vi "flattenVelocityToXML_Scalar.vi"(8 "error in (no error)":errorcluster, 9 "velocityUnitInXML":T1, 10 "velocityAgain":variant, 11 "velocity":dbl[unit]) -> (0 "error out":errorcluster, 3 "xmlString":string)   [LabVIEW 2016, in "UnitsAndXML.lvlib"]
uses:
  <userlib>/Common/UnitsAndXML/UnitsAndXML.lvlib
  <userlib>/Common/UnitsAndXML/FlattenItemWithUnitToXML/FlattenVelocityToXML/VelocityUnit.ctl
  <vilib>/Utility/VariantDataType/VariantType.lvlib
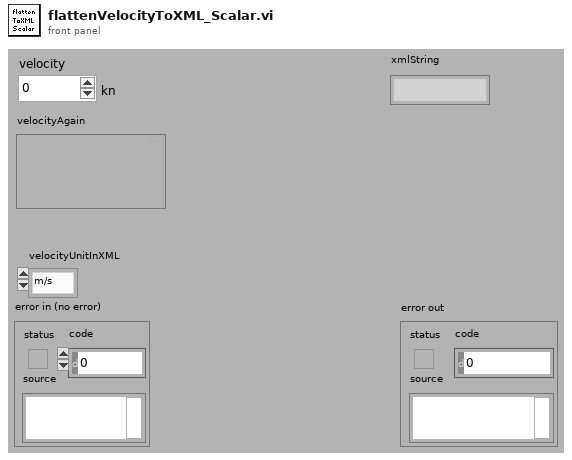
[diagram p1: front panel]
types:
  T1 = typedef "UnitsAndXML.lvlib/VelocityUnit.ctl" = enum16{"m/s", "km/s", "kn"}
  T2 = typedef "VariantType.lvlib/Type.ctl" = enum8{"Invalid Type", "Void", "I8", "I16", "I32", "I64", "U8", "U16", "U32", "U64", "Single Float", "Double Float", "Extended Float", "Single Complex", "Double Complex", "Extended Complex", "Enum U8", "Enum U16", "Enum U32", "Enum U64", "Single Float With Unit", "Double Float With Unit", "Extended Float With Unit", "Single Complex with Unit", "Double Complex with Unit", "Extended Complex with Unit", "Boolean", "String", "Path", "Picture", "Tag", "Array", "Cluster", "Variant", "LV Variant", "Waveform", "Timestamp", "Digital Waveform", "Digital Data", "ExpressData", "Refnum", "External Data", "VI", "Poly VI", "LabVIEW Class Instance", "Fixed Point"}
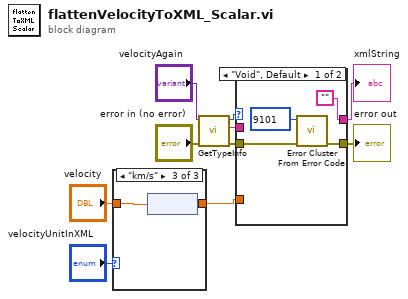
[diagram p0: block diagram]
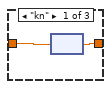
[diagram p2: hidden frame]
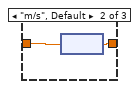
[diagram p3: hidden frame]
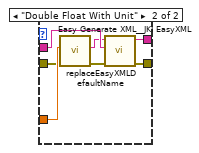
[diagram p4: hidden frame]
diagram:
  n1 = case shown="\"km/s\"" "velocityUnitInXML" {
    tunnel: "velocity" -> [w12 w14 w16]
    tunnel: [w11 w13 w15] -> w2
    frame "kn" {
      n2 = node(w12) -> (w11:dbl)
    }
    frame "m/s", Default {
      n3 = node(w14) -> (w13:dbl)
    }
    frame "km/s" {
      n4 = node(w16) -> (w15:dbl)
    }
  }
  n5 = call <vilib>:"GetTypeInfo.vi"("error in (no error)"="error in (no error)", "Variant"="velocityAgain") -> ("error out"=w5:errorcluster, "Name"=w4:string, "Type Enum"=w6:T2)  [unwired: 5 in, 2 out]
  n6 = case shown="\"Void\", Default" w6 {
    tunnel: w2 -> [_ w27]
    tunnel: ["" w26] -> w10
    tunnel: [w19 w25] -> w9
    tunnel: w5 -> [w17 w22]
    tunnel: w4 -> [_ w24]
    frame "Void", Default {
      n7 = call <vilib>:"Error Cluster From Error Code.vi"("error in (no error)"=w17, "error code (0)"=9101) -> ("error out"=w19:errorcluster)  [unwired: 7 in]
    }
    frame "Double Float With Unit" {
      n8 = call <vilib>:"Easy Generate XML__JKI EasyXML.vi"("error in (no error)"=w22, "LabVIEW Data"=w27) -> ("error out"=w21:errorcluster, "XML String"=w23:string)  [unwired: 8 in]
      n9 = call <userlib>:"replaceEasyXMLDefaultName.vi"("error in"=w21, "desiredName"=w24, "easyXMLStringWithDefaultNames"=w23) -> ("error out"=w25:errorcluster, "xmlString"=w26:string)  [unwired: 7 in]
    }
  }
  "xmlString" <- w10
  "error out" <- w9
